vi "update_success.vi"(11 "Mission in":refnum<class "Mission.lvclass">) -> (1 "Done?":bool, 3 "Mission out":refnum<class "Mission.lvclass">)   [LabVIEW 2011, in "Mission.lvclass"]
uses:
  Mission.lvclass
  Mission.lvclass/Mission.ctl
  2 Globals/2 Global.vi
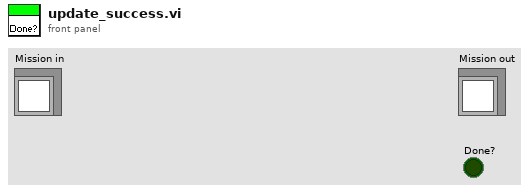
[diagram p1: front panel]
types:
  T1 = enum16{"Round Buoy", "Drive", "Pass Buoys", "Station Keeping"}
  T2 = typedef "Waypoints List.ctl" = refnum<class "Waypoint.lvclass">[]
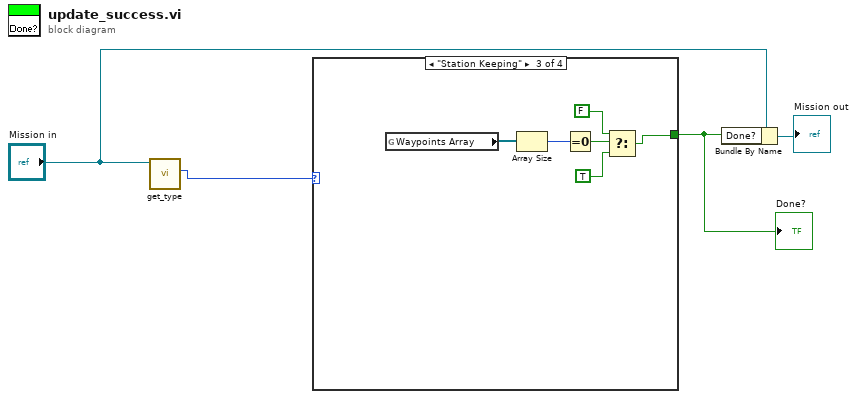
[diagram p0: block diagram]
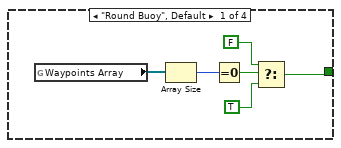
[diagram p2: hidden frame]
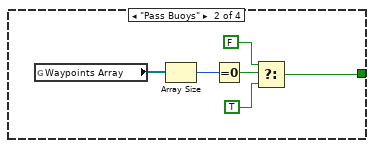
[diagram p3: hidden frame]
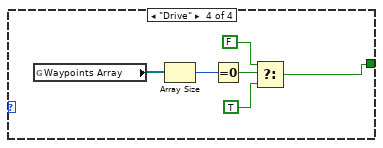
[diagram p4: hidden frame]
diagram:
  n1 = call-dynamic "get_type.vi"("Mission in"="Mission in") -> ("Mission Type"=w1:T1)  [unwired: 8 in, 2 out]
  n2 = case shown="\"Station Keeping\"" w1 {
    tunnel: [w5 w11 w17 w23] -> w2
    frame "Round Buoy", Default {
      n3 = global read "2 Global.vi" "Waypoints Array"() -> (w10:T2)
      n4 = Array Size(array=w10) -> (size(s)=w9:i32)
      n5 = Equal To 0?(x=w9) -> (x = 0?=w7:bool)
      n6 = Select(t=FALSE, s=w7, f=TRUE) -> (s? t:f=w5:bool)
    }
    frame "Pass Buoys" {
      n7 = global read "2 Global.vi" "Waypoints Array"() -> (w16:T2)
      n8 = Array Size(array=w16) -> (size(s)=w15:i32)
      n9 = Equal To 0?(x=w15) -> (x = 0?=w13:bool)
      n10 = Select(t=FALSE, s=w13, f=TRUE) -> (s? t:f=w11:bool)
    }
    frame "Station Keeping" {
      n11 = global read "2 Global.vi" "Waypoints Array"() -> (w22:T2)
      n12 = Array Size(array=w22) -> (size(s)=w21:i32)
      n13 = Equal To 0?(x=w21) -> (x = 0?=w19:bool)
      n14 = Select(t=FALSE, s=w19, f=TRUE) -> (s? t:f=w17:bool)
    }
    frame "Drive" {
      n15 = global read "2 Global.vi" "Waypoints Array"() -> (w28:T2)
      n16 = Array Size(array=w28) -> (size(s)=w27:i32)
      n17 = Equal To 0?(x=w27) -> (x = 0?=w25:bool)
      n18 = Select(t=FALSE, s=w25, f=TRUE) -> (s? t:f=w23:bool)
    }
  }
  "Done?" <- w2
  n19 = Bundle By Name(cluster="Mission in", "Done?"=w2) -> (→"Mission out":refnum<class "Mission.lvclass">)
